vi "Configure Logic Trigger.vi"(0 "VISA resource name":refnum<visa-resource-name>, 9 "Holdoff Type(0: Time)":u16(ring) items=["Time", "Events", "None"], 11 "error in (no error)":errorcluster, 12 "Holdoff Value by Time (50ns)":dbl=5e-08, 14 "Holdoff Value by Events (1)":i32=1) -> (4 "VISA resource name out":refnum<visa-resource-name>, 15 "error out":errorcluster)   [LabVIEW 2020, in "LeCroy Wave Series.lvlib"]
doc: "Configures logic trigger settings. Logic trigger enables triggering on a logical combination (pattern) of five inputs: CH1, CH2, CH3, CH4, EXT. You have a choice of four Boolean operators (AND, NAND, OR, NOR), and you can stipulate the high or low voltage logic level for each input independently.\nTo configure the logical combination of inputs, use lcwave Configure Trigger Pattern.vi."
uses:
  LeCroy Wave Series.lvlib
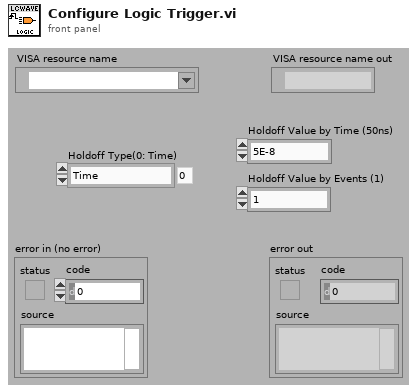
[diagram p1: front panel]
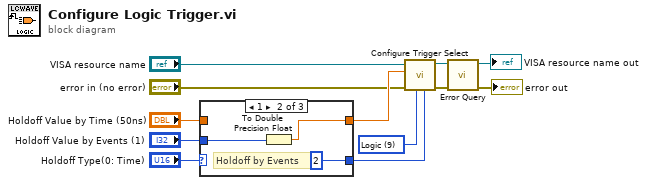
[diagram p0: block diagram]
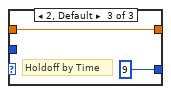
[diagram p3: hidden frame]
diagram:
  w3 = u16 9 items=["Edge", "Dropout", "Glitch", "Interval", "Std", "Sng", "State Qualify", "Edge Qualify", "Width", "Logic"] ("Trigger type")
  n1 = case shown="1" "Holdoff Type(0: Time)" {
    selector: "Holdoff Type(0: Time)" -> [w13 _ _]
    tunnel: [w14 w15 w19] -> w10
    tunnel: "Holdoff Value by Time (50ns)" -> [w14 _ w19]
    tunnel: "Holdoff Value by Events (1)" -> [_ w16 _]
    tunnel: [w13 2 9] -> w6
    frame 0 {
    }
    frame 1 {
      # "Holdoff by Events"
      n2 = To Double Precision Float(number=w16) -> (double precision float=w15:dbl)
    }
    frame 2, Default {
      # "Holdoff by Time"
    }
  }
  n3 = call "Configure Trigger Select.vi"("Hold Type (0: TI)"=w6, "Trigger type"=w3, "error in (no error)"="error in (no error)", "Hold Value 1 (4 ns)"=w10, "VISA resource name"="VISA resource name") -> ("error out"=w1:errorcluster, "VISA resource name out"=w2:refnum<visa-resource-name>)  [unwired: 5 in]
  n4 = call "Error Query.vi"("error in (no error)"=w1, "VISA resource name"=w2) -> ("error out"=→"error out":errorcluster, "VISA resource name out"=→"VISA resource name out":refnum<visa-resource-name>)  [unwired: 6 in, 2 out]
